vi "Initialize.vi"(8 "Error In":errorcluster, 11 "libssh2-lv Shared Library In":path=path "") -> (0 "Error Out":errorcluster={"status"=TRUE, "code"=13, "source"="Call Library Function Node in LabSSH2.lvlib:Initialize.vi->Tests.lvlib:Initialize-Shutdown.vi"}, 3 "libssh2-lv Shared Library Out":path=path "D:/Users/cfield/Code/Field R&D Services/SSH/LabSSH2/LabVIEW/trunk/src/LabSSH2/Private/labssh2.*")   [LabVIEW 2017, in "Toolkit.lvlib"]
uses:
  Toolkit.lvlib
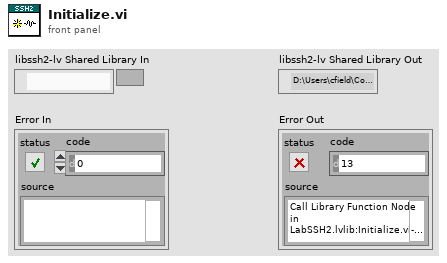
[diagram p1: front panel]
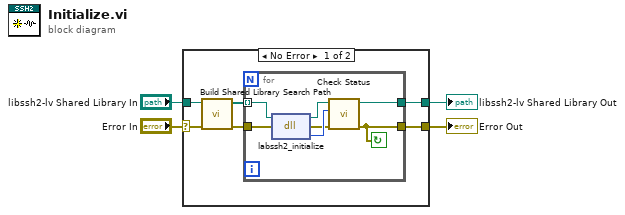
[diagram p0: block diagram]
diagram:
  n1 = case shown="No Error" "Error In" {
    selector: "Error In" -> [w10 w18]
    tunnel: "libssh2-lv Shared Library In" -> [w9 _]
    tunnel: [w5 w18] -> w2
    tunnel: [w6 _] -> w1
    frame No Error {
      n2 = call "Build Shared Library Search Path.vi"("Error In"=w10, "labssh2 Shared Library"=w9) -> ("Error Out"=w7:errorcluster, "Search Path"=w8:path[])  [unwired: 8 in]
      n3 = for {
        tunnel: w8 -> [w16] mode=indexing
        tunnel: w7 -> [w17]
        tunnel: [w14] -> w6
        tunnel: [w11] -> w5
        stop <- w11 continue-if-true
        n4 = dll-call lib="D:/Users/cfield/Code/Field R&D Services/SSH/LabSSH2/LabVIEW/trunk/src/Toolkit/Support/labssh2.*" fn="labssh2_initialize"(path in=w16, error in=w17) -> (path out=w15:path, error out=w12:errorcluster, "return type"=w13:i32)  [unwired: 1 in]
        n5 = call "Check Status.vi"("Error In"=w12, "Status"=w13, "labssh2 Shared Library In"=w15) -> ("Error Out"=w11:errorcluster, "labssh2 Shared Library Out"=w14:path)  [unwired: 7 in]
      }
    }
    frame Error {
    }
  }
  "Error Out" <- w2
  "libssh2-lv Shared Library Out" <- w1
